vi "Set HTTP Port.vi"(8 "error in (no error)":errorcluster, 10 "HTTP Port":u16, 11 "Node in":refnum<class "Node.lvclass">) -> (0 "error out":errorcluster, 3 "Node out":refnum<class "Node.lvclass">)   [LabVIEW 2020, in "VolatusConfig.lvlib" / "Node.lvclass"]
uses:
  Node.lvclass
  C:/dev/lv20CE/relink/lv-volatus/VolatusConfig/VolatusConfigElement/VolatusConfigElement.lvclass
  VolatusConfigElement/VolatusConfigElement.lvclass/VolatusConfigElement.ctl
  lv-cdm/CDM-Config/Config Element/Write Variant Value.vi
  Node.lvclass/Node.ctl
  VolatusConfigElement/VolatusConfigElement.lvclass
  lv-cdm/CDM-Config/Config Element/Config Element.lvclass
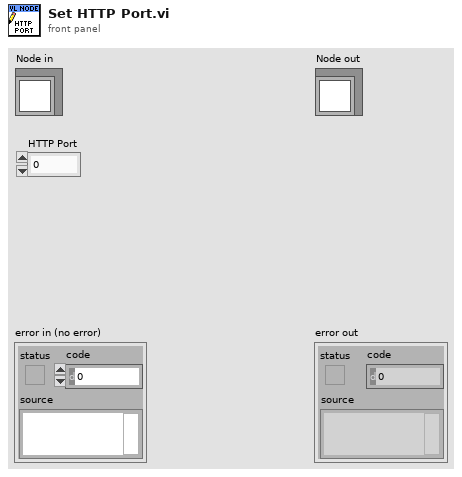
[diagram p1: front panel]
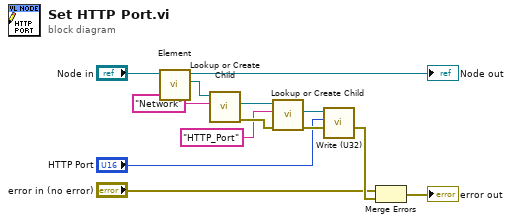
[diagram p0: block diagram]
diagram:
  n1 = call "Element.vi"("VolatusConfigElement in"="Node in") -> ("Element"=w12:refnum<class "Config Element.lvclass">, "VolatusConfigElement out"=→"Node out":refnum<class "Node.lvclass">)  [unwired: 9 in]
  n2 = call "Lookup or Create Child.vi"("Name"="Network", "Config Element in"=w12) -> ("error out"=w13:errorcluster, "Child"=w10:refnum<class "Config Element.lvclass">)  [unwired: 6 in, 2 out]
  n3 = call "Lookup or Create Child.vi"("error in (no error)"=w13, "Name"="HTTP_Port", "Config Element in"=w10) -> ("error out"=w7:errorcluster, "Child"=w8:refnum<class "Config Element.lvclass">)  [unwired: 5 in, 2 out]
  n4 = call "Write (U32).vi"("error in (no error)"=w7, "U32 Value"="HTTP Port", "Config Element in"=w8) -> ("error out"=w6:errorcluster)  [unwired: 7 in, 1 out]
  n5 = Merge Errors("error in (no error)", w6) -> (→"error out":errorcluster)
